vi "SetUser.vi"(8 "error in (no error)":errorcluster, 10 "User":string, 11 "SequenceRun in":refnum<class "SequenceRun.lvclass">) -> (0 "error out":errorcluster, 3 "SequenceRun out":refnum<class "SequenceRun.lvclass">)   [LabVIEW 2021, in "ProligentXMLGenerator.lvlib" / "SequenceRun.lvclass"]
doc: "Defines the user that executed the sequence run.\n\nThis attribute cannot be updated."
uses:
  SequenceRun.lvclass
  SequenceRun.lvclass/SequenceRun.ctl
  Base/Attribute/Attribute.lvclass
  Base/NonEmptyString_255/NonEmptyString_255.lvclass
  C:/Projects/proligent-xml-generator-labview/src/ProligentXMLGenerator/Base/NonEmptyString/NonEmptyString.lvclass
  C:/Projects/proligent-xml-generator-labview/src/ProligentXMLGenerator/Base/String/String.lvclass
  C:/Projects/proligent-xml-generator-labview/src/ProligentXMLGenerator/Base/Attribute/Attribute.lvclass
  C:/Projects/proligent-xml-generator-labview/src/ProligentXMLGenerator/Base/NonEmptyString_255/NonEmptyString_255.lvclass
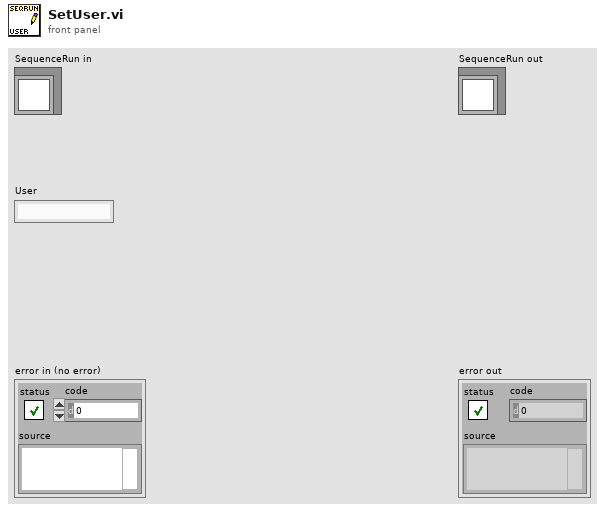
[diagram p1: front panel]
types:
  T1 = typedef "ProligentXMLGenerator.lvlib/SequenceRun.lvclass/Data.ctl" = cluster{"Name":string, "StepRuns":refnum<class "StepRun.lvclass">[], "Characteristics":refnum<class "Characteristic.lvclass">[], "Documents":refnum<class "Document.lvclass">[], "FailureReferences":refnum<class "FailureReference.lvclass">[], "CustomData":refnum<class "CustomData.lvclass">, "StartDate":refnum<class "DateTime.lvclass">, "EndDate":refnum<class "DateTime.lvclass">, "SequenceExecutionStatus":refnum<class "ExecutionStatus.lvclass">, "SequenceRunId":refnum<class "Guid.lvclass">, "SequenceFullName":refnum<class "SequenceFullName.lvclass">, "SequenceVersion":refnum<class "NonEmptyString_64.lvclass">, "StationFullName":refnum<class "FullName.lvclass">, "User":refnum<class "NonEmptyString_255.lvclass">, "TimeZoneInfoId":string}
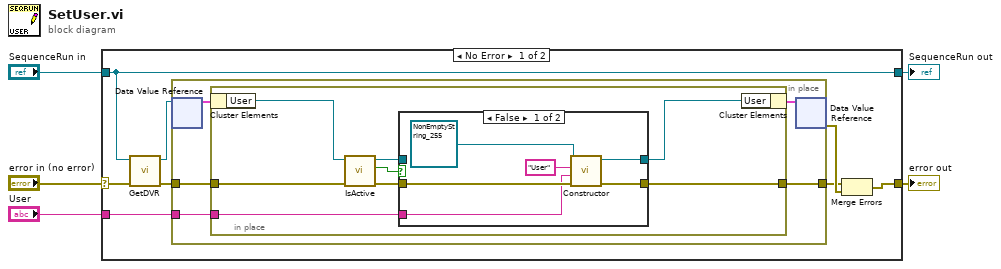
[diagram p0: block diagram]
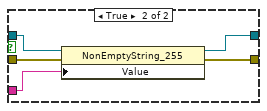
[diagram p2: hidden frame]
diagram:
  n1 = case shown="No Error" "error in (no error)" {
    selector: "error in (no error)" -> [w11 w38]
    tunnel: "SequenceRun in" -> [w6 w39]
    tunnel: [w8 w38] -> w2
    tunnel: "User" -> [w7 _]
    tunnel: [w6 w39] -> w3
    frame No Error {
      n2 = call "GetDVR.vi"("error in"=w11, "SequenceRun"=w6) -> ("error out"=w10:errorcluster, "DVRReference"=w12:refnum<data-value>)  [unwired: 8 in]
      n3 = in-place "In Place Element Structure" {
        in-place-border: w10 -> [w18]
        in-place-border: [w17] -> w9
        in-place-border: w7 -> [w16]
        n4 = in-place-dvr #1(w12) -> (w15:T1)  [unwired: 1 out]
        n5 = in-place "In Place Element Structure" {
          in-place-border: w18 -> [w22]
          in-place-border: [w26] -> w17
          in-place-border: w16 -> [w25]
          n6 = in-place-cluster #2(w15) -> ("User"=w21:refnum<class "NonEmptyString_255.lvclass">)
          n7 = call "IsActive.vi"("error in"=w22, "Attribute in"=w21) -> ("error out"=w23:errorcluster, "IsActive"=w19:bool, "Attribute in"=w20:refnum<class "NonEmptyString_255.lvclass">)  [unwired: 7 in]
          n8 = case shown="False" w19 {
            tunnel: w23 -> [w29 w37]
            tunnel: [w32 w36] -> w26
            tunnel: w25 -> [w28 w35]
            tunnel: [w31 w34] -> w24
            tunnel: w20 -> [_ w33]
            frame False {
              n9 = call-dynamic "Constructor.vi"("error in"=w29, "Value"=w28, "Name"="User", "String in"=refnum<class "NonEmptyString_255.lvclass"> refnum ("ProcessVersion")) -> ("error out"=w32:errorcluster, "String out"=w31:refnum<class "NonEmptyString_255.lvclass">)  [unwired: 6 in]
            }
            frame True {
              n10 = property on="Property Node" class="NonEmptyString_255"(reference=w33, error in=w37, "Value"=w35) -> (reference out=w34:refnum<class "NonEmptyString_255.lvclass">, error out=w36:errorcluster)
            }
          }
          n11 = in-place-cluster #2("User"=w24) -> (w14:T1)
        }
        n12 = in-place-dvr #1(w14) -> (w13:errorcluster)  [unwired: 1 out]
      }
      n13 = Merge Errors(w9, w13) -> (w8:errorcluster)
    }
    frame Error {
    }
  }
  "error out" <- w2
  "SequenceRun out" <- w3
